vi "stop_message_vmc.vi"(10 "notifier":refnum<notifier>) -> (2 "退出命令":string, 3 "Exit？":bool)   [LabVIEW 2012]
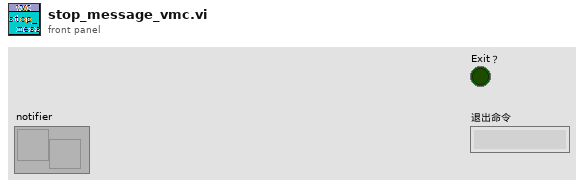
[diagram p1: front panel]
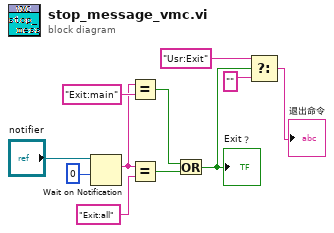
[diagram p0: block diagram]
diagram:
  n1 = Wait on Notification(notifier="notifier", timeout in ms (-1)=0 ("超时毫秒(-1)")) -> (notification=w8:string)  [unwired: 2 in, 3 out]
  n2 = Equal?(x=w8, y="Exit:main") -> (x = y?=w6:bool)
  n3 = Equal?(x=w8, y="Exit:all") -> (x = y?=w7:bool)
  n4 = Or(x=w6, y=w7) -> (x .or. y?=w5:bool)
  "Exit？" <- w5
  n5 = Select(t="Usr:Exit" ("y"), s=w5, f="") -> (s? t:f=→"退出命令":string)
